vi "Test Split Range.vi"(8 "error in (no error)":errorcluster, 11 "Test Case In":refnum<class "Tests.lvclass">) -> (0 "error out":errorcluster, 3 "Test Case Out":refnum<class "Tests.lvclass">)   [LabVIEW 2021, in "Tests.lvclass"]
uses:
  Tests.lvclass
  C:/Program Files (x86)/National Instruments/LabVIEW 2021/vi.lib/Astemes/LUnit/Test Case.lvclass
  Proto/xmas.ctl
  <vilib>/Astemes/LUnit/Test Case.lvclass/Test Case.ctl
  4993e8ee-a06a-463a-9684-69129f64d5ce.vi
  <vilib>/Astemes/LUnit/Append Pass Result.vi
  <vilib>/Astemes/LUnit/Append Fail Result.vi
  <vilib>/Astemes/LUnit/Compare Variants.vi
  <vilib>/Astemes/LUnit/Describe Comparison of Arrays.vi
  <vilib>/Astemes/LUnit/Variant to string.vi
  <vilib>/AdvancedString/1D String Array to Delimited String.vi
  <vilib>/Utility/Data Type/Get Type Information.vi
  <vilib>/Utility/LVClass/Get LV Class Name.vi
  Tests.lvclass/Tests.ctl
  Proto/Rule.lvclass
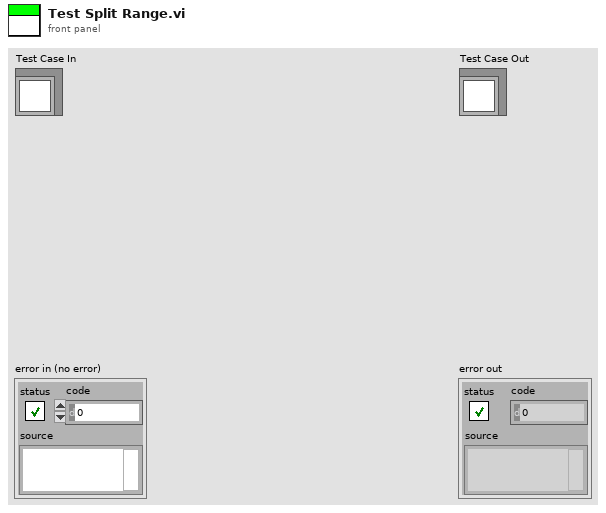
[diagram p1: front panel]
types:
  T1 = typedef "xmas.ctl" = cluster{"from":cluster{"x":u64, "m":u64, "a":u64, "s":u64}, "to":cluster{"x":u64, "m":u64, "a":u64, "s":u64}}
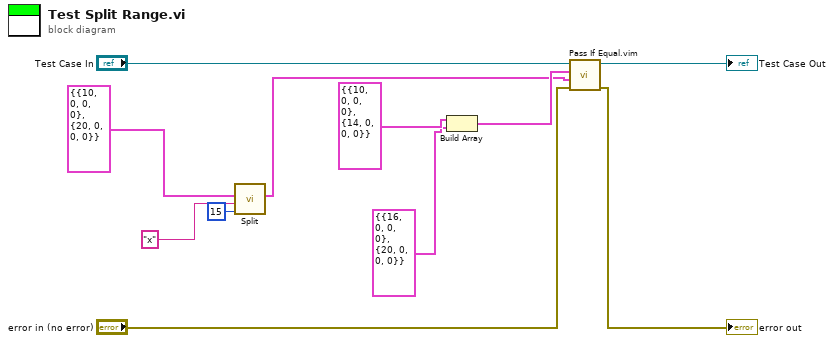
[diagram p0: block diagram]
diagram:
  n1 = call "Split.vi"("Val"=15, "Label"="x", "Cluster"=T1 {"from"={"x"=10, "m"=0, "a"=0, "s"=0}, "to"={"x"=20, "m"=0, "a"=0, "s"=0}}) -> ("Result"=w1:T1[])  [unwired: 8 in]
  n2 = Build Array(T1 {"from"={"x"=10, "m"=0, "a"=0, "s"=0}, "to"={"x"=14, "m"=0, "a"=0, "s"=0}} ("Cluster"), T1 {"from"={"x"=16, "m"=0, "a"=0, "s"=0}, "to"={"x"=20, "m"=0, "a"=0, "s"=0}} ("Cluster")) -> (w2:T1[])
  n3 = call "Pass If Equal.vim"("error in (no error)"="error in (no error)", "Actual"=w1, "Expected"=w2, "LUnit Test Case In"="Test Case In") -> ("error out"=→"error out":errorcluster, "LUnit Test Case Out"=→"Test Case Out":refnum<class "Tests.lvclass">)  [unwired: 6 in]
